vi "Measure.vi"(8 "error in (no error)":errorcluster, 10 "Time in ms (30000)":i32=30000, 11 "VISA resource name":refnum<visa-resource-name>) -> (0 "error out":errorcluster, 2 "output":dbl[](array[numeric]), 3 "VISA resource name out":refnum<visa-resource-name>)   [LabVIEW 2014, in "GP22_TDC_Arduinoed.lvlib"]
doc: "Measure the time between triggers and output an array of all these measurements in the given measurement period."
uses:
  GP22_TDC_Arduinoed.lvlib
  Private/ConvertTimes - Array.vi
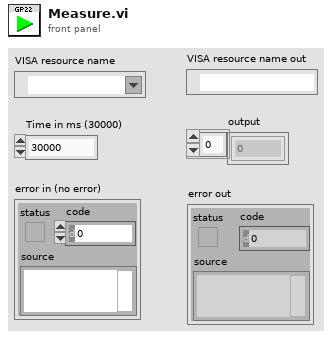
[diagram p1: front panel]
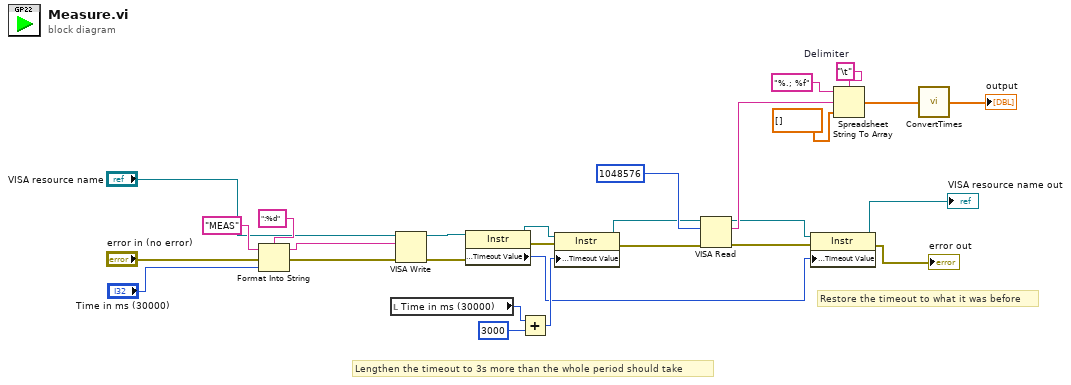
[diagram p0: block diagram]
diagram:
  w20 = "\t"  # Delimiter
  # "Restore the timeout to what it was before"
  # "Lengthen the timeout to 3s more than the whole period should take"
  n1 = Format Into String(format string=":%d", initial string="MEAS" ("command"), error in="error in (no error)", "Time in ms (30000)") -> (resulting string=w22:string, error out=w26:errorcluster)
  n2 = local read "Time in ms (30000)"() -> (w9:i32)
  n3 = VISA Write(VISA resource name="VISA resource name", write buffer=w22, error in (no error)=w26) -> (VISA resource name out=w16:refnum<visa-resource-name>, error out=w15:errorcluster)  [unwired: 1 out]
  n4 = property class="Instr"(reference=w16, error in=w15) -> (reference out=w14:refnum<visa-resource-name>, error out=w13:errorcluster, "General Settings:Timeout Value"=w3:u32)
  n5 = Add(x=w9, y=3000) -> (x+y=w10:i32)
  n6 = property class="Instr"(reference=w14, error in=w13, "General Settings:Timeout Value"=w10) -> (reference out=w12:refnum<visa-resource-name>, error out=w11:errorcluster)
  n7 = VISA Read(VISA resource name=w12, byte count=u32 1048576, error in (no error)=w11) -> (VISA resource name out=w7:refnum<visa-resource-name>, read buffer=w17:string, error out=w6:errorcluster)  [unwired: 1 out]
  n8 = property class="Instr"(reference=w7, error in=w6, "General Settings:Timeout Value"=w3) -> (reference out=→"VISA resource name out":refnum<visa-resource-name>, error out=→"error out":errorcluster)
  n9 = Spreadsheet String To Array(delimiter (Tab)=w20, format string="%.; %f", spreadsheet string=w17, array type (2D Dbl)=dbl[] []) -> (array=w2:dbl[])
  n10 = call-poly "ConvertTimes.vi"("GP22 results"=w2) -> ("Array of times / s"=→"output":dbl[])
